vi "Execute.vi"(8 "error in":errorcluster, 10 "Shifted Error in":refnum<class "Error.lvclass">, 11 "ERROR_Add UUT Error in":refnum<class "ERROR_Add UUT Error.lvclass">) -> (0 "error out":errorcluster, 1 "STOP?":bool, 2 "Shifted Error out":refnum<class "Error.lvclass">, 3 "ERROR_Add UUT Error out":refnum<class "ERROR_Add UUT Error.lvclass">)   [LabVIEW 2019, in "TSC Error.lvlib" / "ERROR_Add UUT Error.lvclass"]
doc: "This Message sets the UUT's Custom Error path location - that can be read and included for errors inserted into an application.\n\nInputs:\n-Error in [obj] - the dynamic dispatch input class\n-Shifted Error in [obj] - the shifted error class with shared information in the Error Loop\n-error in\n\nOutputs:\n-Error out [obj] - the dynamic dispatch output class\n-Shifted Error in [obj] - the shifted error class with shared information\n-STOP? [Boolean] - the output Boolean used to stop the Error Loop\n-error out\n\n<b>Code Developed By:</b>\nDaniel Coons\nTechnology Service Corporation\n1983 S Liberty Drive\nBloomington, IN 47403\nPhone: 812 558-7100\nwww.tsc.com\\atcs"
uses:
  ERROR_Add UUT Error.lvclass
  C:/Development/Open Source/tsc-error-library/_Messages/Error/Error.lvclass
  Error/Error.lvclass
  Error/Error.lvclass/Error.ctl
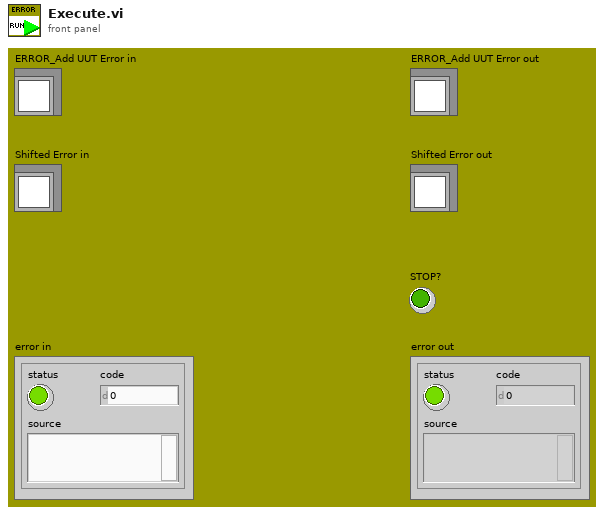
[diagram p1: front panel]
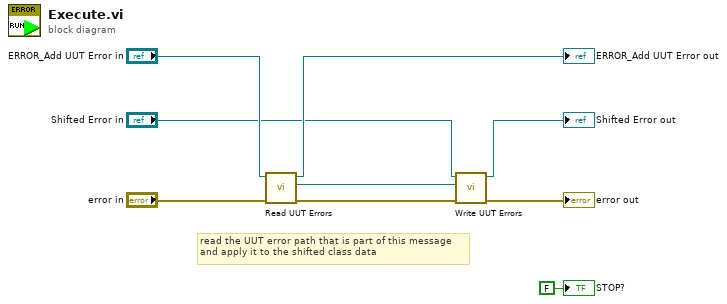
[diagram p0: block diagram]
diagram:
  # "read the UUT error path that is part of this message\nand apply it to the shifted class data"
  n1 = call "Read UUT Errors.vi"("error in (no error)"="error in", "Error in"="ERROR_Add UUT Error in") -> ("error out"=w6:errorcluster, "UUT Errors"=w3:path, "Error out"=→"ERROR_Add UUT Error out":refnum<class "ERROR_Add UUT Error.lvclass">)  [unwired: 7 in]
  n2 = call "Write UUT Errors.vi"("error in (no error)"=w6, "UUT Errors"=w3, "Error in"="Shifted Error in") -> ("error out"=→"error out":errorcluster, "Error out"=→"Shifted Error out":refnum<class "Error.lvclass">)  [unwired: 7 in]
  "STOP?" <- FALSE ("STOP?")
